vi "correctornombre.vi"(10 "NUEVA":string) -> (2 "concatenated string":string)   [LabVIEW 2016]
panel:
  out "Array":i32[](array[numeric])
  out "offset past match":i32
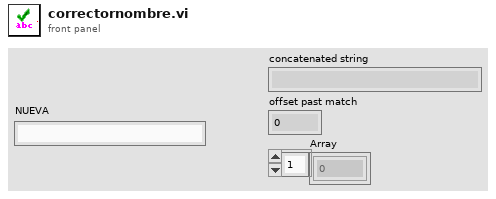
[diagram p1: front panel]
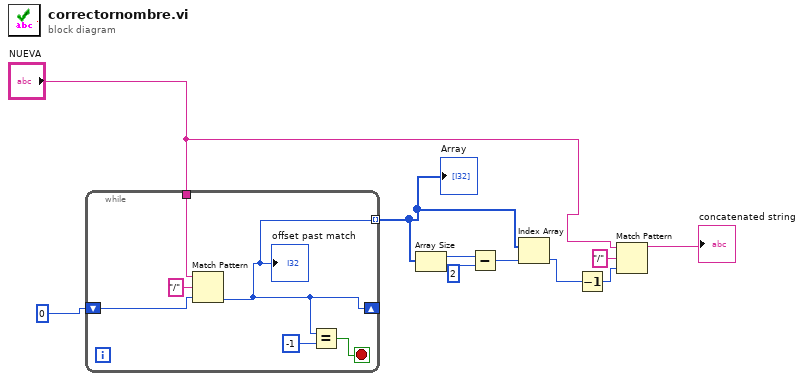
[diagram p0: block diagram]
diagram:
  n1 = while {
    tunnel: "NUEVA" -> [w15]
    shift-right: [w11] -> _
    shift-left: 0 -> [w12]
    tunnel: [w11] -> w2 mode=indexing
    stop <- w14 stop-if-true
    n2 = Match Pattern(string=w15, regular expression="/", offset (0)=w12) -> (offset past match=w11:i32)  [unwired: 3 out]
    "offset past match" <- w11
    n3 = Equal?(x=w11, y=-1) -> (x = y?=w14:bool)
  }
  "Array" <- w2
  n4 = Array Size(array=w2) -> (size(s)=w9:i32)
  n5 = Subtract(x=w9, y=2) -> (x-y=w3:i32)
  n6 = Index Array(array=w2, index=w3) -> (element=w1:i32)
  n7 = Decrement(x=w1) -> (x-1=w5:i32)
  n8 = Match Pattern(string="NUEVA", regular expression="/", offset (0)=w5) -> (before substring=→"concatenated string":string)  [unwired: 3 out]
